vi "Set Connection Status.vi"(8 "error in (no error)":errorcluster, 9 "connected?":bool, 10 "Connection Status":T1, 11 "IP Connection in":refnum<class "IP Connection.lvclass">) -> (0 "error out":errorcluster, 3 "IP Connection out":refnum<class "IP Connection.lvclass">)   [LabVIEW 2011, in "Tinkerforge.lvlib" / "IP Connection.lvclass"]
doc: "This VI sets the connection status of the IP Connection."
uses:
  IP Connection.lvclass
  Type Definitions/Connection Status.ctl
  IP Connection.lvclass/IP Connection.ctl
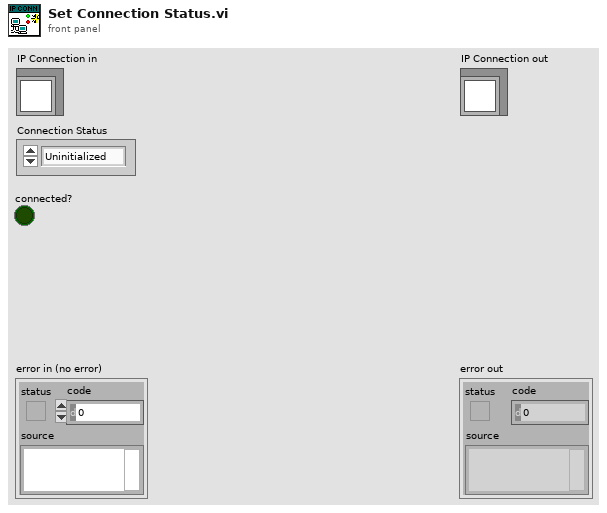
[diagram p1: front panel]
types:
  T1 = typedef "Tinkerforge.lvlib/IP Connection.lvclass/Connection Status.ctl" = enum16{"Uninitialized", "Connected", "Reconnecting", "Disconnected"}
  T2 = typedef "Tinkerforge.lvlib/IP Connection.lvclass/Connection.ctl" = cluster{"TCP Network Connection":refnum<k5>, "is connected":bool, "Connection Status":T1}
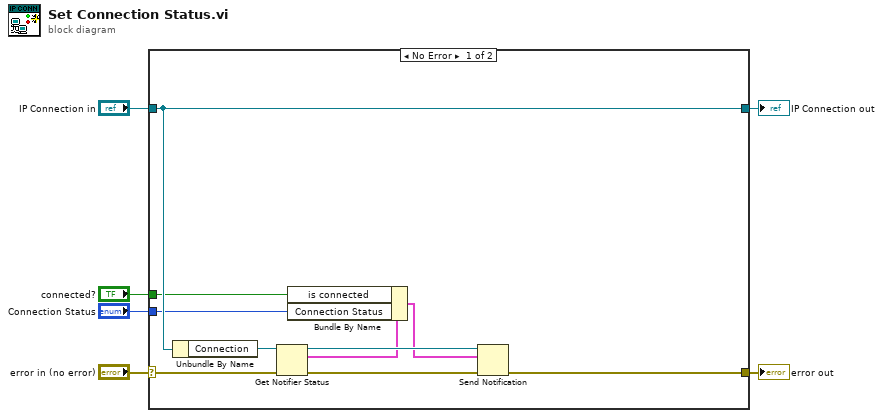
[diagram p0: block diagram]
diagram:
  n1 = case shown="No Error" "error in (no error)" {
    selector: "error in (no error)" -> [w10 w18]
    tunnel: [w14 w18] -> w5
    tunnel: [w16 w17] -> w3
    tunnel: "IP Connection in" -> [w16 w17]
    tunnel: "connected?" -> [w13 _]
    tunnel: "Connection Status" -> [w12 _]
    frame No Error {
      n2 = Unbundle By Name(w16) -> ("Connection"=w15:refnum<notifier>)
      n3 = Get Notifier Status(notifier=w15, error in (no error)=w10) -> (notifier out=w11:refnum<notifier>, current notification=w8:T2, error out=w9:errorcluster)  [unwired: 2 out]
      n4 = Bundle By Name(cluster=w8, "is connected"=w13, "Connection Status"=w12) -> (w7:T2)
      n5 = Send Notification(notification=w7, notifier=w11, error in (no error)=w9) -> (error out=w14:errorcluster)  [unwired: 1 out]
    }
    frame Error {
    }
  }
  "error out" <- w5
  "IP Connection out" <- w3
